vi "Lift Cases.vi"() -> ()   [LabVIEW 2014]
uses:
  Begin/Global Variables.vi
panel:
  in  "mult":dbl=0.7 format="%#_13g"
  in  "Lift Speed Slow idle":dbl=0.6
  in  "Lift Speed Fast":dbl=0.75
  in  "Pickup":dbl=32.0 format="%#_13g"
  in  "Tote 2 Height":dbl=24.0 format="%#_13g"
  in  "Tote 2 Height New":dbl=44.0
  in  "Tote 1 Height New":dbl=7.0
  in  "Tote 3 Height New":dbl=44.0
  in  "Tote 1 Height":dbl=7.5
  in  "Tote 3 Height":dbl=45.5
  in  "Lift Speed":dbl=0.95 format="%#_13g"
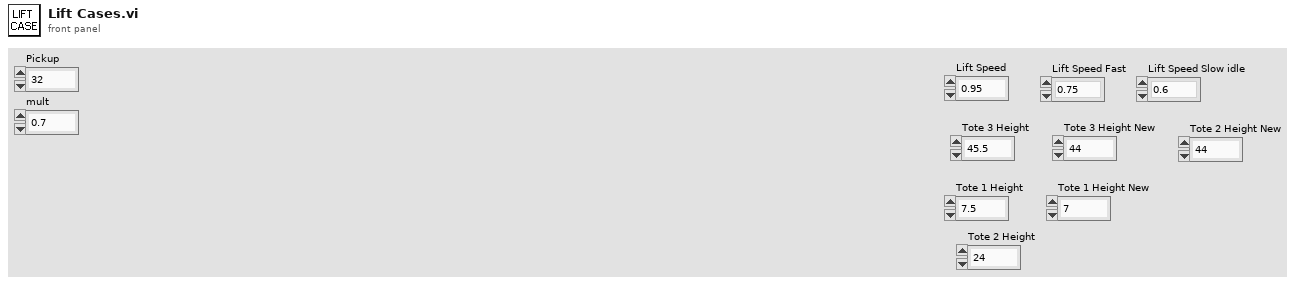
[diagram p1: front panel]
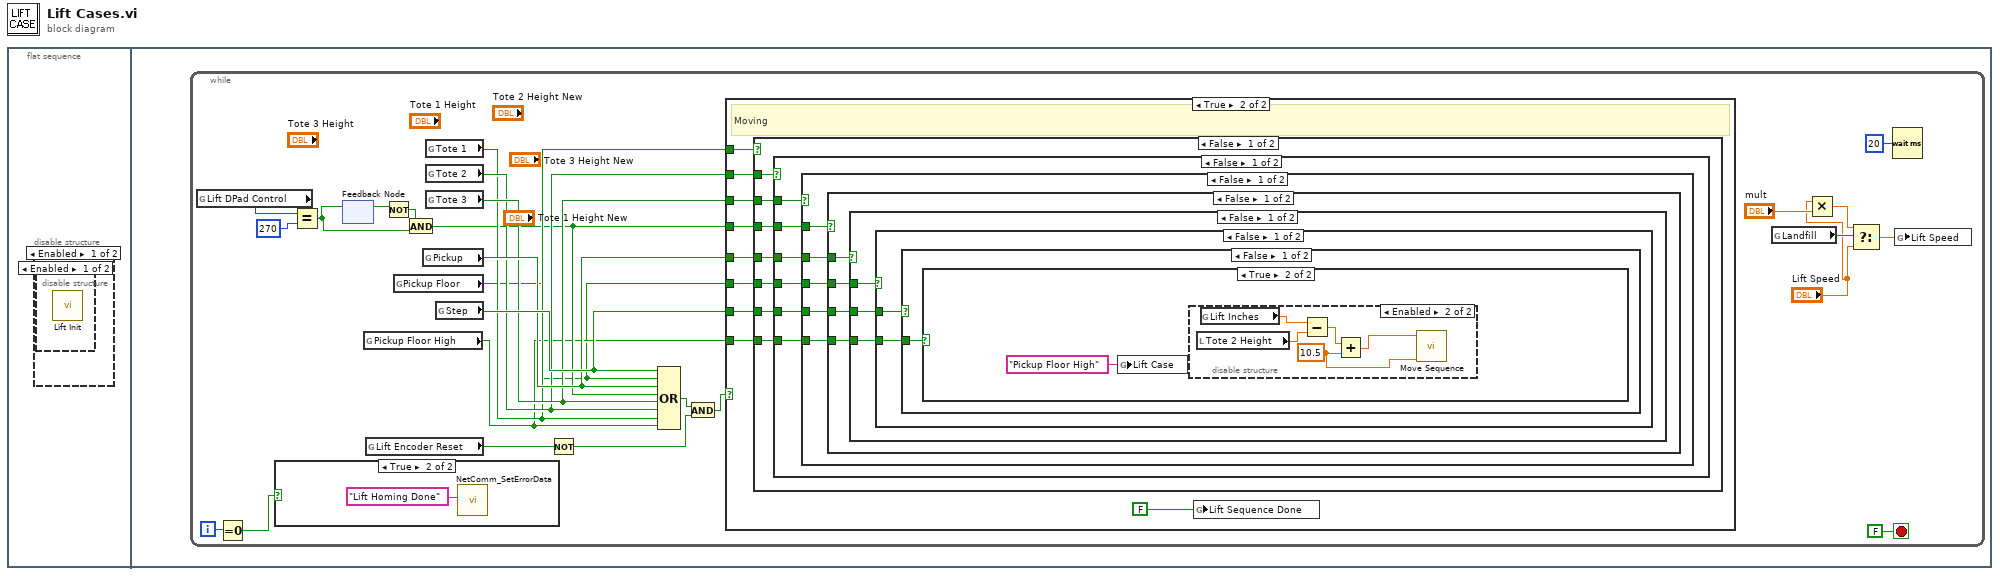
[diagram p0: block diagram]
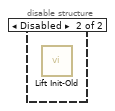
[diagram p2: hidden frame]
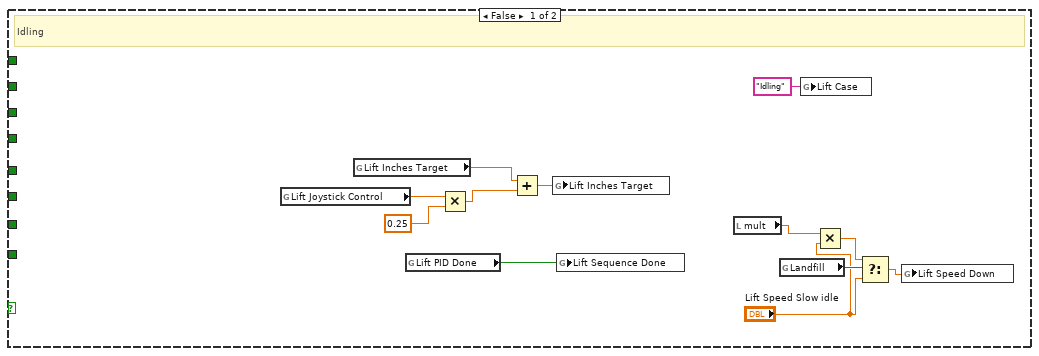
[diagram p5: hidden frame]
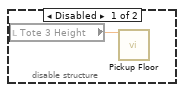
[diagram p7: hidden frame]
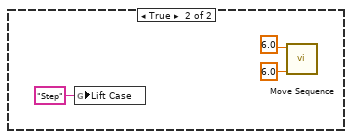
[diagram p8: hidden frame]
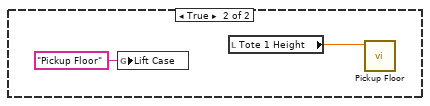
[diagram p9: hidden frame]
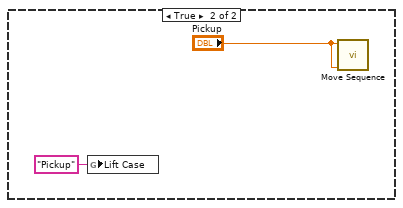
[diagram p10: hidden frame]
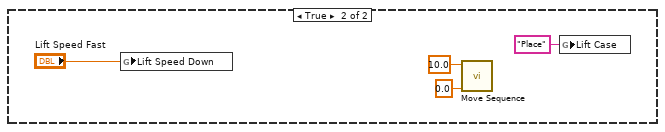
[diagram p11: hidden frame]
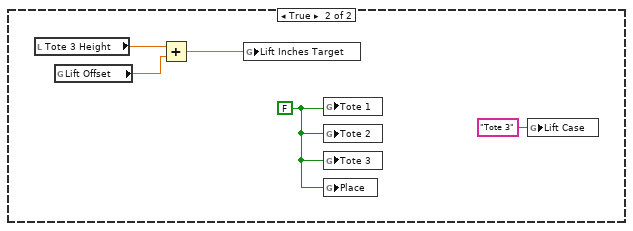
[diagram p12: hidden frame]
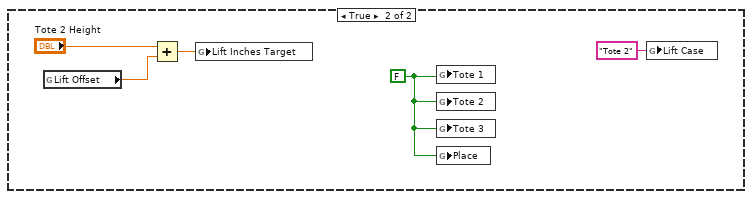
[diagram p13: hidden frame]
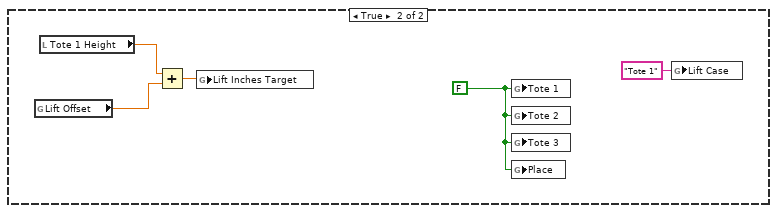
[diagram p14: hidden frame]
diagram:
  n1 = flat-sequence {
    frame #0 {
      n2 = disable-structure shown="Enabled" {
        frame Enabled {
          n3 = disable-structure shown="Enabled" {
            frame Enabled {
              n4 = call "Lift Init.vi"() -> ()  [unwired: 12 in]
            }
            frame Disabled {
              n5 = call "Lift Init-Old.vi"() -> ()  [unwired: 12 in]
            }
          }
        }
        frame Disabled {
        }
      }
    }
    frame #1 {
      n6 = while {
        i -> [w2]
        stop <- FALSE stop-if-true
        n7 = global read "Global Variables.vi" "Lift DPad Control"() -> (w13:i16)
        n8 = Equal To 0?(x=w2) -> (x = 0?=w1:bool)
        n9 = case shown="True" w1 {
          frame False {
          }
          frame True {
            n10 = call <vilib>:"NetComm_SetErrorData.vi"("Error Data"="Lift Homing Done") -> ()  [unwired: 3 in, 8 out]
          }
        }
        n11 = Equal?(x=w13, y=i16 270) -> (x = y?=w18:bool)
        n12 = feedback #1() -> (w17:bool)  [unwired: 1 in]
        n13 = feedback-in #1(w18) -> ()
        n14 = global read "Global Variables.vi" "Pickup Floor High"() -> (w12:bool)
        n15 = global read "Global Variables.vi" "Lift Encoder Reset"() -> (w20:bool)
        n16 = Not(x=w17) -> (.not. x?=w16:bool)
        n17 = global read "Global Variables.vi" "Pickup Floor"() -> (w10:bool)
        n18 = And(x=w16, y=w18) -> (x .and. y?=w14:bool)
        n19 = global read "Global Variables.vi" "Pickup"() -> (w24:bool)
        n20 = global read "Global Variables.vi" "Tote 1"() -> (w21:bool)
        n21 = global read "Global Variables.vi" "Tote 2"() -> (w22:bool)
        n22 = global read "Global Variables.vi" "Tote 3"() -> (w23:bool)
        n23 = global read "Global Variables.vi" "Step"() -> (w25:bool)
        n24 = Not(x=w20) -> (.not. x?=w19:bool)
        n25 = Compound Arithmetic op=OR(w25, w10, w24, w14, w23, w22, w21, w12) -> (w9:bool)
        n26 = And(x=w9, y=w19) -> (x .and. y?=w8:bool)
        n27 = case shown="True" w8 {
          tunnel: w21 -> [_ w48]
          tunnel: w22 -> [_ w47]
          tunnel: w23 -> [_ w46]
          tunnel: w14 -> [_ w45]
          tunnel: w24 -> [_ w44]
          tunnel: w10 -> [_ w43]
          tunnel: w25 -> [_ w42]
          tunnel: w12 -> [_ w40]
          frame False {
            # "Idling"
            n28 = global read "Global Variables.vi" "Lift Joystick Control"() -> (w35:dbl)
            n29 = global read "Global Variables.vi" "Lift Inches Target"() -> (w37:dbl)
            n30 = global read "Global Variables.vi" "Lift PID Done"() -> (w39:bool)
            n31 = Multiply(x=w35, y=0.25) -> (x*y=w36:dbl)
            n32 = Add(x=w37, y=w36) -> (x+y=w38:dbl)
            n33 = global write "Global Variables.vi" "Lift Inches Target"(w38) -> ()
            n34 = global write "Global Variables.vi" "Lift Sequence Done"(w39) -> ()
            n35 = local read "mult"() -> (w30:dbl)
            n36 = global read "Global Variables.vi" "Landfill"() -> (w33:bool)
            n37 = global write "Global Variables.vi" "Lift Case"("Idling" ("Lift Case")) -> ()
            n38 = Multiply(x=w30, y="Lift Speed Slow idle") -> (x*y=w32:dbl)
            n39 = Select(t=w32, s=w33, f="Lift Speed Slow idle") -> (s? t:f=w31:dbl)
            n40 = global write "Global Variables.vi" "Lift Speed Down"(w31) -> ()
          }
          frame True {
            # "Moving"
            n41 = case shown="False" w48 {
              tunnel: w47 -> [w55 _]
              tunnel: w46 -> [w54 _]
              tunnel: w45 -> [w53 _]
              tunnel: w44 -> [w52 _]
              tunnel: w43 -> [w51 _]
              tunnel: w42 -> [w50 _]
              tunnel: w40 -> [w49 _]
              frame False {
                n42 = case shown="False" w55 {
                  tunnel: w54 -> [w61 _]
                  tunnel: w53 -> [w60 _]
                  tunnel: w52 -> [w59 _]
                  tunnel: w51 -> [w58 _]
                  tunnel: w50 -> [w57 _]
                  tunnel: w49 -> [w56 _]
                  frame False {
                    n43 = case shown="False" w61 {
                      tunnel: w60 -> [w66 _]
                      tunnel: w59 -> [w65 _]
                      tunnel: w58 -> [w64 _]
                      tunnel: w57 -> [w63 _]
                      tunnel: w56 -> [w62 _]
                      frame False {
                        n44 = case shown="False" w66 {
                          tunnel: w65 -> [w70 _]
                          tunnel: w64 -> [w69 _]
                          tunnel: w63 -> [w68 _]
                          tunnel: w62 -> [w67 _]
                          frame False {
                            n45 = case shown="False" w70 {
                              tunnel: w69 -> [w73 _]
                              tunnel: w68 -> [w72 _]
                              tunnel: w67 -> [w71 _]
                              frame False {
                                n46 = case shown="False" w73 {
                                tunnel: w72 -> [w75 _]
                                tunnel: w71 -> [w74 _]
                                frame False {
                                n47 = case shown="False" w75 {
                                tunnel: w74 -> [w76 _]
                                frame False {
                                n48 = case shown="True" w76 {
                                frame False {
                                }
                                frame True {
                                n49 = global write "Global Variables.vi" "Lift Case"("Pickup Floor High" ("Lift Case")) -> ()
                                n50 = disable-structure shown="Enabled" {
                                frame Disabled {
                                n51 = local read "Tote 3 Height"() -> (w78:dbl)
                                n52 = call "Pickup Floor.vi"("Final Height"=w78) -> ()  [unwired: 11 in]
                                }
                                frame Enabled {
                                w79 = 10.5 ("y")
                                n53 = local read "Tote 2 Height"() -> (w82:dbl)
                                n54 = global read "Global Variables.vi" "Lift Inches"() -> (w83:dbl)
                                n55 = Subtract(x=w83, y=w82) -> (x-y=w81:dbl)
                                n56 = Add(x=w81, y=w79) -> (x+y=w80:dbl)
                                n57 = call "Move Sequence.vi"("Distance Up"=w79, "Distance Down"=w80) -> ()  [unwired: 10 in]
                                }
                                }
                                }
                                }
                                }
                                frame True {
                                n58 = global write "Global Variables.vi" "Lift Case"("Step" ("Lift Case")) -> ()
                                n59 = call "Move Sequence.vi"("Distance Up"=6.0, "Distance Down"=6.0) -> ()  [unwired: 10 in]
                                }
                                }
                                }
                                frame True {
                                n60 = global write "Global Variables.vi" "Lift Case"("Pickup Floor" ("Lift Case")) -> ()
                                n61 = local read "Tote 1 Height"() -> (w88:dbl)
                                n62 = call "Pickup Floor.vi"("Final Height"=w88) -> ()  [unwired: 11 in]
                                }
                                }
                              }
                              frame True {
                                n63 = global write "Global Variables.vi" "Lift Case"("Pickup" ("Lift Case")) -> ()
                                n64 = call "Move Sequence.vi"("Distance Up"="Pickup", "Distance Down"="Pickup") -> ()  [unwired: 10 in]
                              }
                            }
                          }
                          frame True {
                            n65 = global write "Global Variables.vi" "Lift Speed Down"("Lift Speed Fast") -> ()
                            n66 = call "Move Sequence.vi"("Distance Up"=0.0, "Distance Down"=10.0 ("Distance Down 2")) -> ()  [unwired: 10 in]
                            n67 = global write "Global Variables.vi" "Lift Case"("Place" ("Lift Case")) -> ()
                          }
                        }
                      }
                      frame True {
                        w97 = FALSE ("Tote 0")
                        n68 = local read "Tote 3 Height"() -> (w96:dbl)
                        n69 = global read "Global Variables.vi" "Lift Offset"() -> (w98:dbl)
                        n70 = Add(x=w96, y=w98) -> (x+y=w99:dbl)
                        n71 = global write "Global Variables.vi" "Lift Inches Target"(w99) -> ()
                        n72 = global write "Global Variables.vi" "Tote 1"(w97) -> ()
                        n73 = global write "Global Variables.vi" "Tote 2"(w97) -> ()
                        n74 = global write "Global Variables.vi" "Tote 3"(w97) -> ()
                        n75 = global write "Global Variables.vi" "Place"(w97) -> ()
                        n76 = global write "Global Variables.vi" "Lift Case"("Tote 3" ("Lift Case")) -> ()
                      }
                    }
                  }
                  frame True {
                    w101 = FALSE ("Tote 0")
                    n77 = global read "Global Variables.vi" "Lift Offset"() -> (w102:dbl)
                    n78 = Add(x="Tote 2 Height", y=w102) -> (x+y=w103:dbl)
                    n79 = global write "Global Variables.vi" "Lift Inches Target"(w103) -> ()
                    n80 = global write "Global Variables.vi" "Tote 1"(w101) -> ()
                    n81 = global write "Global Variables.vi" "Tote 2"(w101) -> ()
                    n82 = global write "Global Variables.vi" "Tote 3"(w101) -> ()
                    n83 = global write "Global Variables.vi" "Place"(w101) -> ()
                    n84 = global write "Global Variables.vi" "Lift Case"("Tote 2" ("Lift Case")) -> ()
                  }
                }
              }
              frame True {
                w107 = FALSE ("Tote 0")
                n85 = global read "Global Variables.vi" "Lift Offset"() -> (w108:dbl)
                n86 = local read "Tote 1 Height"() -> (w106:dbl)
                n87 = Add(x=w106, y=w108) -> (x+y=w109:dbl)
                n88 = global write "Global Variables.vi" "Lift Inches Target"(w109) -> ()
                n89 = global write "Global Variables.vi" "Tote 1"(w107) -> ()
                n90 = global write "Global Variables.vi" "Tote 2"(w107) -> ()
                n91 = global write "Global Variables.vi" "Tote 3"(w107) -> ()
                n92 = global write "Global Variables.vi" "Place"(w107) -> ()
                n93 = global write "Global Variables.vi" "Lift Case"("Tote 1" ("Lift Case")) -> ()
              }
            }
            n94 = global write "Global Variables.vi" "Lift Sequence Done"(FALSE ("Lift Sequence Done")) -> ()
          }
        }
        n95 = global read "Global Variables.vi" "Landfill"() -> (w7:bool)
        n96 = Multiply(x="Lift Speed", y="mult") -> (x*y=w4:dbl)
        n97 = Select(t=w4, s=w7, f="Lift Speed") -> (s? t:f=w6:dbl)
        n98 = Wait (ms)(milliseconds to wait=u32 20) -> ()  [unwired: 1 out]
        n99 = global write "Global Variables.vi" "Lift Speed"(w6) -> ()
      }
    }
  }
